vi "graph surrounding object distance.vi"(9 "point":cluster{"x":i16, "y":i16}, 10 "raster image":bool[][](array[boolean]), 11 "sample resolution":i32) -> (1 "scale multiplier":dbl step=7.75483175952187e-304, 2 "Waveform Graph":sgl[](graph))   [LabVIEW 2009]
panel:
  out "progress":dbl(slide) step=1.9188242573772974e-137 scale=0.0..1.0
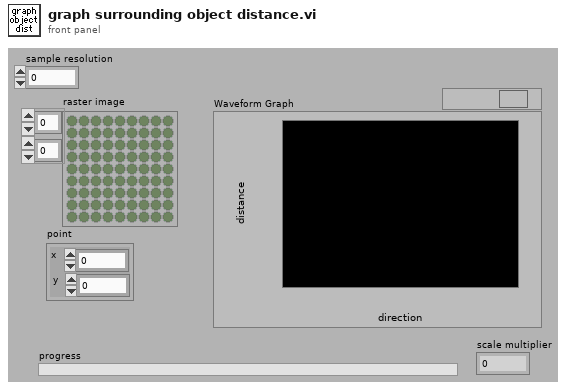
[diagram p1: front panel]
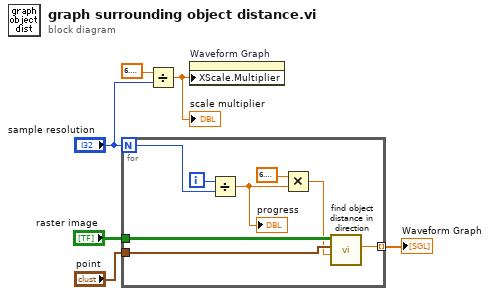
[diagram p0: block diagram]
diagram:
  n1 = for {
    N: "sample resolution" -> [w10]
    tunnel: "raster image" -> [w14]
    tunnel: "point" -> [w13]
    tunnel: [w12] -> w4 mode=indexing
    i -> [w11]
    n2 = Divide(x=w11, y=w10) -> (x/y=w9:dbl)
    "progress" <- w9
    n3 = Multiply(x=6.283185307179586, y=w9) -> (x*y=w7:dbl)
    n4 = call "find object distance in direction.vi"("direction"=w7, "point"=w13, "raster image"=w14) -> ("distance"=w12:sgl)  [unwired: 8 in]
  }
  "Waveform Graph" <- w4
  n5 = Divide(x=6.283185307179586, y="sample resolution") -> (x/y=w1:dbl)
  "scale multiplier" <- w1
  n6 = property on="Waveform Graph" class="WFGraph (strict)"("XScale.Multiplier"=w1) -> ()  [unwired: 2 in, 2 out]
